vi "UpdateEventHandler.vi"(8 "error in (no error)":errorcluster, 10 "UpdateEvent":string, 11 "VMUI in":refnum<class "VMUI.lvclass">) -> (0 "error out":errorcluster, 2 "Stop":bool, 3 "VMUI out":refnum<class "VMUI.lvclass">)   [LabVIEW 2013, in "VMUI.lvclass"]
uses:
  VMUI.lvclass
  <vilib>/Utility/miscctls.llb/LVRowAndColumnUnsignedTypeDef.ctl
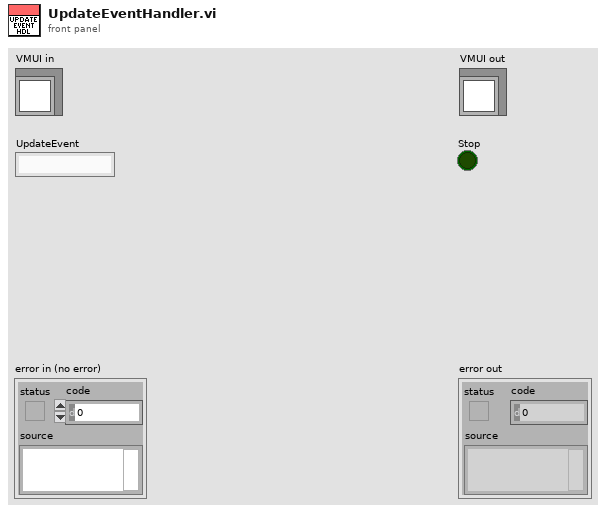
[diagram p1: front panel]
types:
  T1 = typedef "LVRowAndColumnUnsignedTypeDef.ctl" = cluster{"Row":u32, "Column":u32}
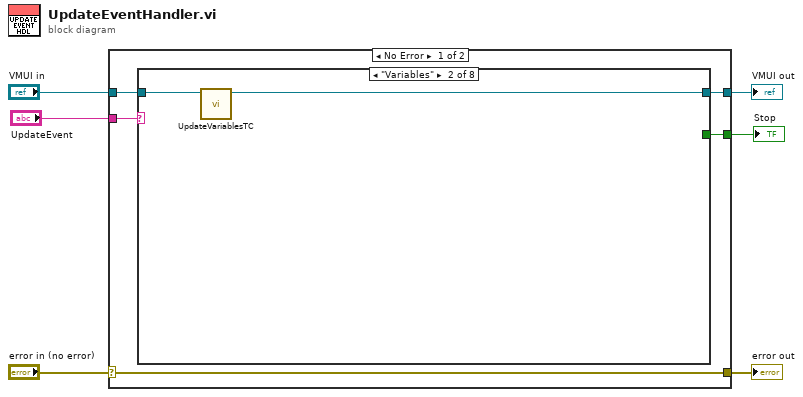
[diagram p0: block diagram]
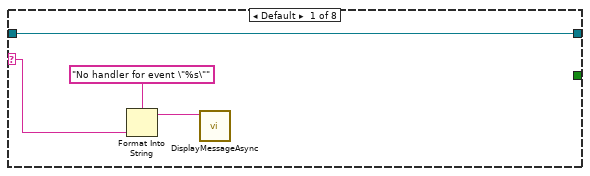
[diagram p2: hidden frame]
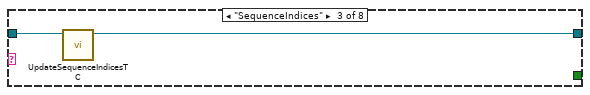
[diagram p3: hidden frame]
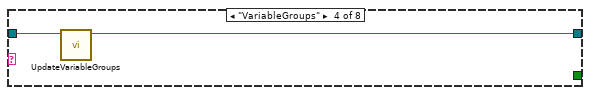
[diagram p4: hidden frame]
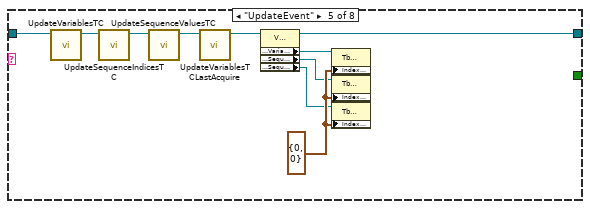
[diagram p5: hidden frame]
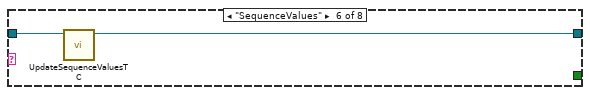
[diagram p6: hidden frame]
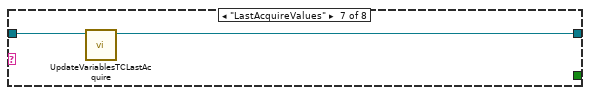
[diagram p7: hidden frame]
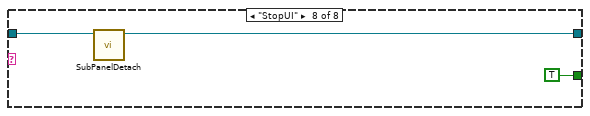
[diagram p8: hidden frame]
diagram:
  n1 = case shown="No Error" "error in (no error)" {
    selector: "error in (no error)" -> [w11 w40]
    tunnel: [w11 w40] -> w5
    tunnel: [w8 w39] -> w3
    tunnel: "VMUI in" -> [w9 w39]
    tunnel: "UpdateEvent" -> [w10 _]
    tunnel: [w7 _] -> w1
    frame No Error {
      n2 = case shown="\"Variables\"" w10 {
        selector: w10 -> [w14 _ _ _ _ _ _ _]
        tunnel: [w12 w16 w18 w20 w25 w32 w34 w36] -> w8
        tunnel: w9 -> [w12 w17 w19 w21 w31 w33 w35 w37]
        tunnel: [_ _ _ _ _ _ _ TRUE] -> w7
        frame Default {
          n3 = Format Into String(format string="No handler for event \"%s\"", w14) -> (resulting string=w13:string)  [unwired: 2 in, 1 out]
          n4 = call "DisplayMessageAsync.vi"("Message"=w13) -> ()  [unwired: 11 in]
        }
        frame "Variables" {
          n5 = call-dynamic "UpdateVariablesTC.vi"("VMUI in"=w17) -> ("VMUI out"=w16:refnum<class "VMUI.lvclass">)  [unwired: 9 in, 1 out]
        }
        frame "SequenceIndices" {
          n6 = call-dynamic "UpdateSequenceIndicesTC.vi"("VMUI in"=w19) -> ("VMUI out"=w18:refnum<class "VMUI.lvclass">)  [unwired: 9 in, 1 out]
        }
        frame "VariableGroups" {
          n7 = call-dynamic "UpdateVariableGroups.vi"("VMUI in"=w21) -> ("VMUI out"=w20:refnum<class "VMUI.lvclass">)  [unwired: 9 in, 1 out]
        }
        frame "UpdateEvent" {
          w27 = T1 {"Row"=0, "Column"=0} ("Index Values")
          n8 = call-dynamic "UpdateVariablesTC.vi"("VMUI in"=w31) -> ("VMUI out"=w30:refnum<class "VMUI.lvclass">)  [unwired: 9 in, 1 out]
          n9 = call-dynamic "UpdateSequenceIndicesTC.vi"("VMUI in"=w30) -> ("VMUI out"=w29:refnum<class "VMUI.lvclass">)  [unwired: 9 in, 1 out]
          n10 = call-dynamic "UpdateSequenceValuesTC.vi"("VMUI in"=w29) -> ("VMUI out"=w28:refnum<class "VMUI.lvclass">)  [unwired: 9 in, 1 out]
          n11 = call-dynamic "UpdateVariablesTCLastAcquire.vi"("VMUI in"=w28) -> ("VMUI out"=w26:refnum<class "VMUI.lvclass">)  [unwired: 9 in, 1 out]
          n12 = property class="VMUI.lvclass"(reference=w26) -> (reference out=w25:refnum<class "VMUI.lvclass">, "Accessors:VariablesTCRef"=w24:refnum<vi>, "Accessors:SequenceIndicesTCRef"=w23:refnum<vi>, "Accessors:SequenceValuesTCRef"=w22:refnum<vi>)  [unwired: 1 in, 1 out]
          n13 = property class="Tbl (strict)"(reference=w24, "Index Values"=w27) -> ()  [unwired: 1 in, 2 out]
          n14 = property class="Tbl (strict)"(reference=w23, "Index Values"=w27) -> ()  [unwired: 1 in, 2 out]
          n15 = property class="Tbl (strict)"(reference=w22, "Index Values"=w27) -> ()  [unwired: 1 in, 2 out]
        }
        frame "SequenceValues" {
          n16 = call-dynamic "UpdateSequenceValuesTC.vi"("VMUI in"=w33) -> ("VMUI out"=w32:refnum<class "VMUI.lvclass">)  [unwired: 9 in, 1 out]
        }
        frame "LastAcquireValues" {
          n17 = call-dynamic "UpdateVariablesTCLastAcquire.vi"("VMUI in"=w35) -> ("VMUI out"=w34:refnum<class "VMUI.lvclass">)  [unwired: 9 in, 1 out]
        }
        frame "StopUI" {
          n18 = call-dynamic "SubPanelDetach.vi"("VMUI in"=w37) -> ("VMUI out"=w36:refnum<class "VMUI.lvclass">)  [unwired: 9 in, 1 out]
        }
      }
    }
    frame Error {
    }
  }
  "error out" <- w5
  "VMUI out" <- w3
  "Stop" <- w1
